vi "Read IA.vi"(8 "error in (no error)":errorcluster, 11 "State Data in":refnum<class "State Data.lvclass">) -> (0 "error out":errorcluster, 2 "IA":cluster{"Mean":dbl, "Error":dbl}[](array[cluster]), 3 "State Data out":refnum<class "State Data.lvclass">)   [LabVIEW 2015, in "State Data.lvclass"]
uses:
  State Data.lvclass
  State Data.lvclass/State Data.ctl
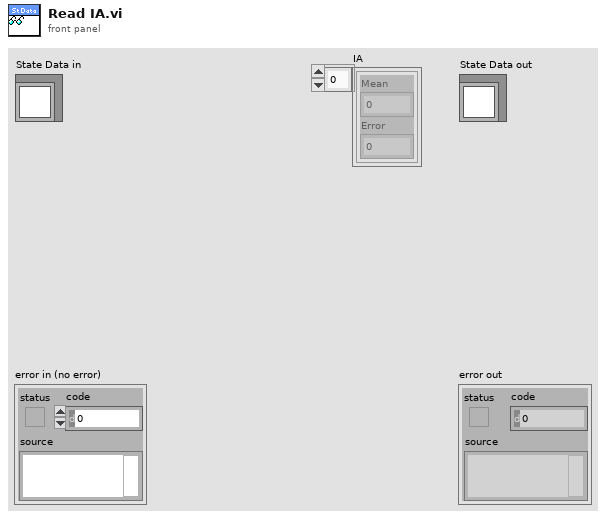
[diagram p1: front panel]
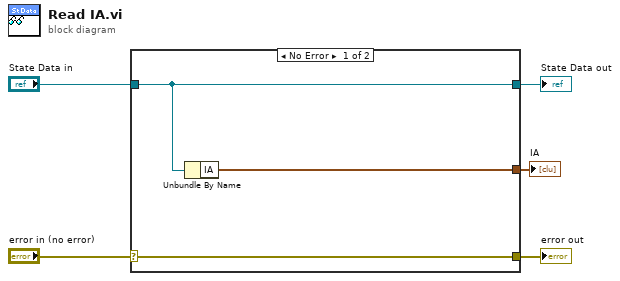
[diagram p0: block diagram]
diagram:
  n1 = case shown="No Error" "error in (no error)" {
    selector: "error in (no error)" -> [w8 w9]
    tunnel: [w8 w9] -> w4
    tunnel: [w7 w10] -> w2
    tunnel: "State Data in" -> [w7 w10]
    tunnel: [w6 _] -> w1
    frame No Error {
      n2 = Unbundle By Name(w7) -> ("IA"=w6:cluster{"Mean":dbl, "Error":dbl}[])
    }
    frame Error {
    }
  }
  "error out" <- w4
  "State Data out" <- w2
  "IA" <- w1
